vi "Trapezodial Velocity Profile.vi"(3 "Final Position":dbl, 4 "Max Velocity":dbl, 5 "Max Acceleration":dbl, 6 "Encoder Refnum":string) -> (0 "Current Position (Setpoint)":dbl, 1 "Current Velocity (Setpoint)":dbl, 2 "Current Acceleration (Setpoint)":dbl)   [LabVIEW 2012]
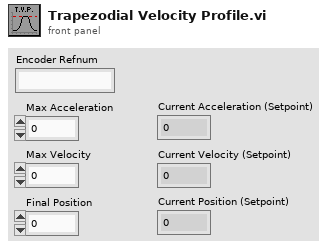
[diagram p1: front panel]
types:
  T1 = typedef "WPI_EncoderDevRef.ctl" = cluster{"DevStatus":errorcluster, "EncoderIndex":T2, "CounterIndex":T3, "DistancePerCount":dbl, "Decoding Type":T4}
  T2 = typedef "FPGA_EncoderIdx.ctl" = enum8{"Enc 0", "Enc 1", "Enc 2", "Enc 3", "Invalid"}
  T3 = typedef "FPGA_CounterCtrSystemIndex.ctl" = enum8{"Ctr 0", "Ctr 1", "Ctr 2", "Ctr 3", "Ctr 4", "Ctr 5", "Ctr 6", "Ctr 7", "Invalid"}
  T4 = typedef "WPI_EncoderType.ctl" = enum16{"1x", "2x", "4x"}
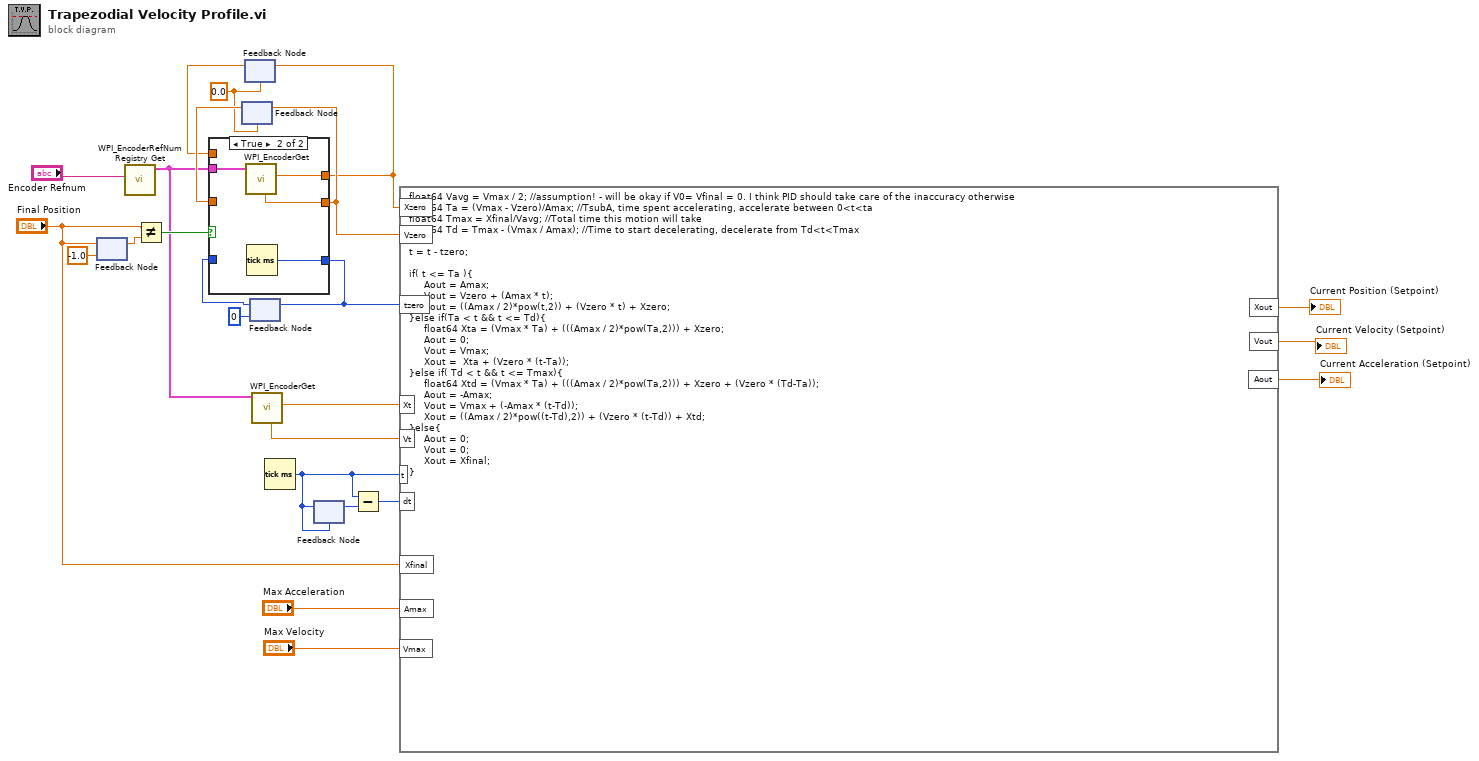
[diagram p0: block diagram]
diagram:
  w3 = 0.0 ("Rate")
  n1 = feedback-in #1("Final Position") -> ()
  n2 = feedback #1(-1.0 ("Final Position")) -> (w23:dbl)
  n3 = call <vilib>:"WPI_EncoderRefNum Registry Get.vi"("refnum name"="Encoder Refnum") -> ("EncoderDevRef"=w11:T1)  [unwired: 9 in, 1 out]
  n4 = Not Equal?(x="Final Position", y=w23) -> (x != y?=w21:bool)
  n5 = feedback #2(w3) -> (w16:dbl)
  n6 = feedback #3(w3) -> (w1:dbl)
  n7 = feedback #4(u32 0 ("millisecond timer value")) -> (w19:u32)
  n8 = case shown="True" w21 {
    tunnel: [w27 w31] -> w18
    tunnel: w19 -> [w27 _]
    tunnel: w11 -> [_ w30]
    tunnel: [w26 w29] -> w15
    tunnel: w16 -> [w26 _]
    tunnel: [w25 w28] -> w2
    tunnel: w1 -> [w25 _]
    frame False {
    }
    frame True {
      n9 = call <vilib>:"WPI_EncoderGet.vi"("EncoderDevRef"=w30) -> ("Distance"=w28:dbl, "Rate"=w29:dbl)  [unwired: 5 in, 4 out]
      n10 = Tick Count (ms)() -> (millisecond timer value=w31:u32)
    }
  }
  n11 = feedback-in #2(w15) -> ()
  n12 = feedback-in #3(w2) -> ()
  n13 = feedback-in #4(w18) -> ()
  n14 = call <vilib>:"WPI_EncoderGet.vi"("EncoderDevRef"=w11) -> ("Distance"=w9:dbl, "Rate"=w10:dbl)  [unwired: 5 in, 4 out]
  n15 = Tick Count (ms)() -> (millisecond timer value=w8:u32)
  n16 = feedback-in #5(w8) -> ()
  n17 = feedback #5(w8) -> (w7:u32)
  n18 = Subtract(x=w8, y=w7) -> (x-y=w6:u32)
  n19 = formula code="float64 Vavg = Vmax / 2; //assumption! - will be okay if V0= Vfinal = 0. I think PID should take care of the inaccuracy otherwise\nfloat64 Ta = (Vmax - Vzero)/Amax; //TsubA, time spent accelerating, accelerate between 0<t<ta\nfloat64 Tmax = Xfinal/Vavg; //Total time this motion will take\nfloat64 Td = Tmax - (Vmax / Amax); //Time to start decelerating, decelerate from Td<t<Tmax\n\nt = t - tzero;\n\nif( t <= Ta ){\n     Aout = Amax;\n     Vout = Vzero + (Amax * t);\n     Xout = ((Amax / 2)*pow(t,2)) + (Vzero * t) + Xzero;\n}else if(Ta < t && t <= Td){\n     float64 Xta = (Vmax * Ta) + (((Amax / 2)*pow(Ta,2))) + Xzero;\n     Aout = 0;\n     Vout = Vmax;\n     Xout =  Xta + (Vzero * (t-Ta));\n}else if( Td < t && t <= Tmax){\n     float64 Xtd = (Vmax * Ta) + (((Amax / 2)*pow(Ta,2))) + Xzero + (Vzero * (Td-Ta));\n     Aout = -Amax;\n     Vout = Vmax + (-Amax * (t-Td));\n     Xout = ((Amax / 2)*pow((t-Td),2)) + (Vzero * (t-Td)) + Xtd;\n}else{\n     Aout = 0;\n     Vout = 0;\n     Xout = Xfinal;\n}"("Xfinal"="Final Position", "tzero"=w18, "Vzero"=w15, "Amax"="Max Acceleration", "Vmax"="Max Velocity", "t"=w8, "Xt"=w9, "Vt"=w10, "dt"=w6, "Xzero"=w2) -> ("Xout"=→"Current Position (Setpoint)":dbl, "Vout"=→"Current Velocity (Setpoint)":dbl, "Aout"=→"Current Acceleration (Setpoint)":dbl)
